vi "Read.vi"(5 "Username":string, 6 "Password":string, 7 "Address":string, 8 "Error In":errorcluster) -> (0 "Error Out":errorcluster)   [LabVIEW 2018, in "Tests.lvlib" / "Channel.lvlib"]
uses:
  Channel.lvlib
  <vilib>/addons/_JKI Toolkits/Caraya/classes/Test/Test.lvclass
  <vilib>/addons/_JKI Toolkits/Caraya/classes/Assert/Assert.lvclass
  src/Toolkit/Channel/Channel.lvclass
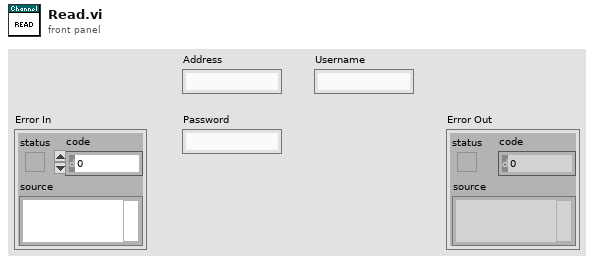
[diagram p1: front panel]
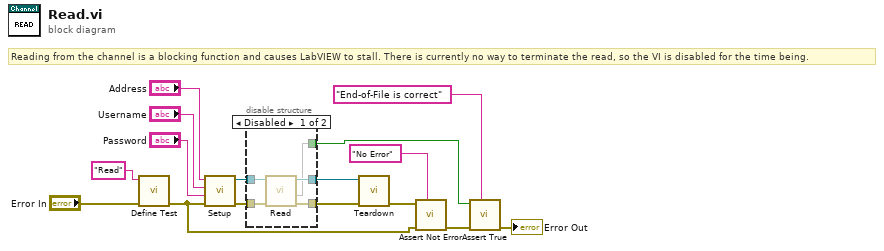
[diagram p0: block diagram]
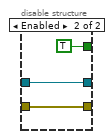
[diagram p2: hidden frame]
diagram:
  # "Reading from the channel is a blocking function and causes LabVIEW to stall. There is currently no way to terminate the read, so the VI is disabled for the time being."
  n1 = call <vilib>:"Define Test.vi"("error in (no error)"="Error In", "Label (VI Title)"="Read") -> ("error out"=w12:errorcluster)  [unwired: 9 in]
  n2 = call "Setup.vi"("Error In"=w12, "Password"="Password", "Username"="Username", "Address"="Address") -> ("Error Out"=w7:errorcluster, "Channel"=w8:refnum<class "Channel.lvclass">)  [unwired: 6 in]
  n3 = disable-structure shown="Disabled" {
    disable-tunnel: w8 -> [w21 w24]
    disable-tunnel: w7 -> [w20 w23]
    disable-tunnel: [w19 w24] -> w6
    disable-tunnel: [w18 w23] -> w5
    disable-tunnel: [w17 TRUE ("True?")] -> w2
    frame Disabled {
      n4 = call "Read.vi"("Error In"=w20, "Channel In"=w21) -> ("Error Out"=w18:errorcluster, 1:w17, "Channel Out"=w19:refnum<class "Channel.lvclass">)  [unwired: 6 in, 1 out]
    }
    frame Enabled {
    }
  }
  n5 = call "Teardown.vi"("Error In"=w5, "Channel"=w6) -> ("Error Out"=w4:errorcluster)  [unwired: 9 in]
  n6 = call <vilib>:"Assert Not Error.vi"("Label"="No Error", "error in (no error)"=w12, "Not Error?"=w4) -> ("error out"=w13:errorcluster)  [unwired: 8 in]
  n7 = call <vilib>:"Assert True.vi"("Label"="End-of-File is correct", "error in (no error)"=w13, "True?"=w2) -> ("error out"=→"Error Out":errorcluster)  [unwired: 8 in]
